vi "Normalize Point.vi"(0 "xmax":dbl, 1 "x":dbl, 2 "Coerce (T)":bool=TRUE, 3 "xmin":dbl) -> (5 "y":dbl)   [LabVIEW 2011]
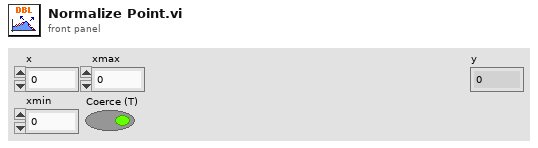
[diagram p1: front panel]
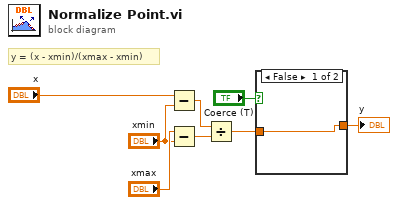
[diagram p0: block diagram]
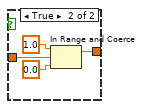
[diagram p2: hidden frame]
diagram:
  # "y = (x - xmin)/(xmax - xmin)"
  n1 = Subtract(x="x", y="xmin") -> (x-y=w7:dbl)
  n2 = Subtract(x="xmax", y="xmin") -> (x-y=w4:dbl)
  n3 = Divide(x=w7, y=w4) -> (x/y=w3:dbl)
  n4 = case shown="False" "Coerce (T)" {
    tunnel: w3 -> [w9 w13]
    tunnel: [w9 w10] -> w2
    frame False {
    }
    frame True {
      n5 = In Range and Coerce(upper limit=1.0, x=w13, lower limit=0.0) -> (coerced(x)=w10:dbl)  [unwired: 1 out]
    }
  }
  "y" <- w2
